vi "specu1a 1.0.0 ProductID-UnitID.vi"(3 "error in":errorcluster, 4 "Unit ID":string, 5 "specu1a 1.0.0 Model Name":T1) -> (0 "error out":errorcluster, 2 "specu1a 1.0.0 Model Name out":T1)   [LabVIEW 2010]
uses:
  Controls/specu1a 1.0.0 Model Class.ctl
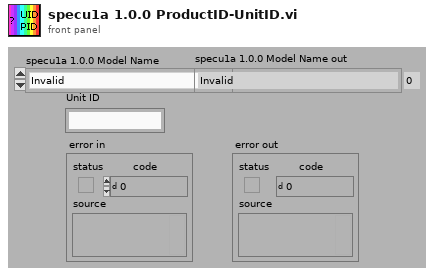
[diagram p1: front panel]
types:
  T1 = typedef "specu1a 1.0.0 Model Class.ctl" = enum16{"Invalid", "TG-NIR or SWNIR or UV", "TG-COOLED NIR-I or II", "TM-UV/VIS or VIS/NIR", "TM-UV/VIS or VIS/NIR CCD1 or CCD2", "RC- Vis or SWNIR Module"}
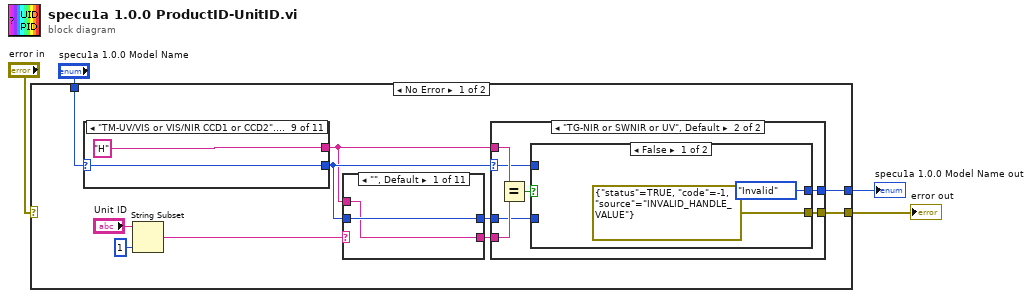
[diagram p0: block diagram]
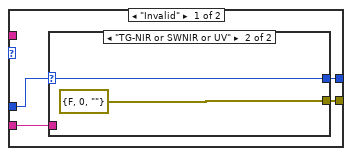
[diagram p2: hidden frame]
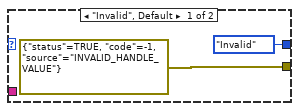
[diagram p3: hidden frame]
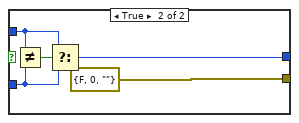
[diagram p4: hidden frame]
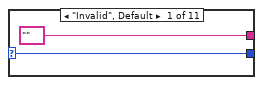
[diagram p5: hidden frame]
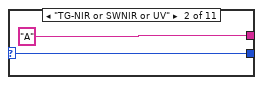
[diagram p6: hidden frame]
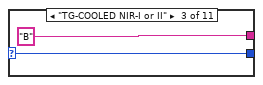
[diagram p7: hidden frame]
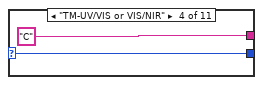
[diagram p8: hidden frame]
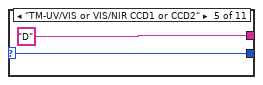
[diagram p9: hidden frame]
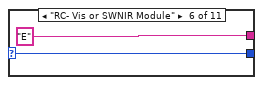
[diagram p10: hidden frame]
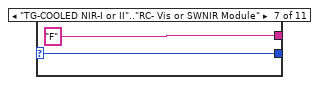
[diagram p11: hidden frame]
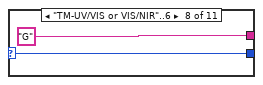
[diagram p12: hidden frame]
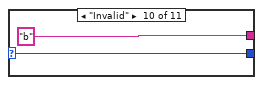
[diagram p13: hidden frame]
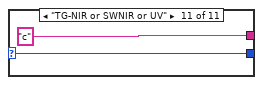
[diagram p14: hidden frame]
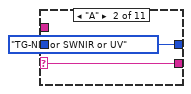
[diagram p15: hidden frame]
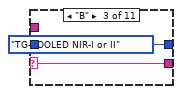
[diagram p16: hidden frame]
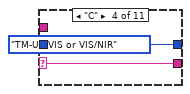
[diagram p17: hidden frame]
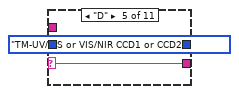
[diagram p18: hidden frame]
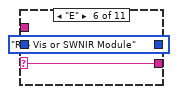
[diagram p19: hidden frame]
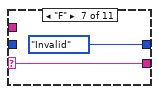
[diagram p20: hidden frame]
diagram:
  n1 = case shown="No Error" "error in" {
    selector: "error in" -> [_ w82]
    tunnel: [w9 w81] -> w4
    tunnel: [w8 w82] -> w3
    tunnel: "specu1a 1.0.0 Model Name" -> [w7 w81]
    frame No Error {
      n2 = case shown="\"TM-UV/VIS-CCD2\"..\"TM-VIS/NIR-CCD2\"" w7 {
        selector: w7 -> [w37 w39 w41 w43 w45 w47 w49 w51 w53 w55 w57]
        tunnel: ["" "A" "B" "C" "D" "E" "F" "G" "H" "b" "c"] -> w5
        tunnel: [w37 w39 w41 w43 w45 w47 w49 w51 w53 w55 w57] -> w6
        frame "Invalid", Default {
        }
        frame "TG-NIR or SWNIR or UV" {
        }
        frame "TG-COOLED NIR-I or II" {
        }
        frame "TM-UV/VIS or VIS/NIR" {
        }
        frame "TM-UV/VIS or VIS/NIR CCD1 or CCD2" {
        }
        frame "RC- Vis or SWNIR Module" {
        }
        frame "TG-COOLED NIR-I or II".."RC- Vis or SWNIR Module" {
        }
        frame "TM-UV/VIS or VIS/NIR"..6 {
        }
        frame "TM-UV/VIS or VIS/NIR CCD1 or CCD2"..7 {
        }
        frame "Invalid" {
        }
        frame "TG-NIR or SWNIR or UV" {
        }
      }
      n3 = String Subset(string="Unit ID", length (rest)=1 ("length (rest)")) -> (substring=w12:string)  [unwired: 1 in]
      n4 = case shown="\"\", Default" w12 {
        selector: w12 -> [_ w61 w63 w65 w67 w69 w71 w73 w75 w77 w79]
        tunnel: [w60 specu1a_1.0.0_Model_Class."TG-NIR or SWNIR or UV" ("specu1a 1.0.0 Model Name") specu1a_1.0.0_Model_Class."TG-COOLED NIR-I or II" ("specu1a 1.0.0 Model Name") specu1a_1.0.0_Model_Class."TM-UV/VIS or VIS/NIR" ("specu1a 1.0.0 Model Name") specu1a_1.0.0_Model_Class."TM-UV/VIS or VIS/NIR CCD1 or CCD2" ("specu1a 1.0.0 Model Name") specu1a_1.0.0_Model_Class."RC- Vis or SWNIR Module" ("specu1a 1.0.0 Model Name") specu1a_1.0.0_Model_Class."Invalid" ("specu1a 1.0.0 Model Name") specu1a_1.0.0_Model_Class."Invalid" ("specu1a 1.0.0 Model Name") specu1a_1.0.0_Model_Class."Invalid" ("specu1a 1.0.0 Model Name") specu1a_1.0.0_Model_Class."Invalid" ("specu1a 1.0.0 Model Name") specu1a_1.0.0_Model_Class."Invalid" ("specu1a 1.0.0 Model Name")] -> w11
        tunnel: [w59 w61 w63 w65 w67 w69 w71 w73 w75 w77 w79] -> w10
        tunnel: w6 -> [w60 _ _ _ _ _ _ _ _ _ _]
        tunnel: w5 -> [w59 _ _ _ _ _ _ _ _ _ _]
        frame "", Default {
        }
        frame "A" {
        }
        frame "B" {
        }
        frame "C" {
        }
        frame "D" {
        }
        frame "E" {
        }
        frame "F" {
        }
        frame "G" {
        }
        frame "H" {
        }
        frame "b" {
        }
        frame "c" {
        }
      }
      n5 = case shown="\"TG-NIR or SWNIR or UV\", Default" w6 {
        selector: w6 -> [_ w25]
        tunnel: w5 -> [_ w29]
        tunnel: w11 -> [w18 w24]
        tunnel: w10 -> [w15 w28]
        tunnel: [w17 w26] -> w8
        tunnel: [w16 w23] -> w9
        frame "Invalid" {
          n6 = case shown="\"TG-NIR or SWNIR or UV\"" w18 {
            selector: w18 -> [_ w22]
            tunnel: [errorcluster {"status"=TRUE, "code"=-1, "source"="INVALID_HANDLE_VALUE"} ("error out") errorcluster {"status"=FALSE, "code"=0, "source"=""} ("error out")] -> w17
            tunnel: [specu1a_1.0.0_Model_Class."Invalid" ("specu1a 1.0.0 Model Name") w22] -> w16
            tunnel: w15 -> [_ _]
            frame "Invalid", Default {
            }
            frame "TG-NIR or SWNIR or UV" {
            }
          }
        }
        frame "TG-NIR or SWNIR or UV", Default {
          n7 = Equal?(x=w29, y=w28) -> (x = y?=w27:bool)
          n8 = case shown="False" w27 {
            tunnel: [errorcluster {"status"=TRUE, "code"=-1, "source"="INVALID_HANDLE_VALUE"} ("error out") errorcluster {"status"=FALSE, "code"=0, "source"=""} ("error out")] -> w26
            tunnel: w25 -> [_ w35]
            tunnel: w24 -> [_ w34]
            tunnel: [specu1a_1.0.0_Model_Class."Invalid" ("specu1a 1.0.0 Model Name") w33] -> w23
            frame False {
            }
            frame True {
              n9 = Not Equal?(x=w35, y=w34) -> (x != y?=w36:bool)
              n10 = Select(t=w35, s=w36, f=w34) -> (s? t:f=w33:T1)
            }
          }
        }
      }
    }
    frame Error {
    }
  }
  "specu1a 1.0.0 Model Name out" <- w4
  "error out" <- w3
